vi "serialization test.vi"() -> ()   [LabVIEW 2013, in "std eng tests.lvlib"]
uses:
  std eng tests.lvlib
  Runtime/Standard Engine Runtime.lvclass
  <vilib>/NI/Tag Bus Module Framework/channel/channel classification.ctl
  <vilib>/NI/Tag Bus/tag/Data Type.ctl
  Configuration/Module Decimation.ctl
  Configuration/Supported Timing Sources.ctl
  testmodule/execution/testmod runtime.lvclass
  testmodule/configuration/testmod configuration.lvclass
  Configuration/Module Error Configuration.ctl
  Configuration/Error Actions By Category.ctl
  <vilib>/NI/Tag Bus Module Framework/runtime/error classification.ctl
  Configuration/Error Actions.ctl
  Configuration/timing reporting tags.ctl
  Configuration/Standard Engine Configuration.lvclass
  Configuration/Standard Engine Configuration.lvclass/Standard Engine Configuration.ctl
  <vilib>/NI/Tag Bus/tag/tag descriptor.lvclass
  Configuration/Write Timing Source Type.vi
  Configuration/Read Master Timing Module.vi
  Configuration/Read Module Specific Configuration.vi
  Configuration/Read Processor.vi
  Configuration/Read timing policy.vi
  Configuration/Read Timing Source Type.vi
  Configuration/Write Timing Source dt.vi
  Configuration/Find Module Specific Config.vi
  <vilib>/Utility/error.llb/Error Cluster From Error Code.vi
  <vilib>/NI/Configuration Framework/error generator.vi
  Configuration/Read Timing Source dt.vi
  <vilib>/NI/Tag Bus Module Framework/channel/TBM channel.lvclass
  <vilib>/NI/Module Execution Interface/Engine Configuration/engine configuration.lvclass
  <vilib>/NI/Tag Bus Module Framework/runtime/TBM module execution interface.lvclass
panel:
  out "Array":T1(array[cluster])
  out "x = y?":T2(array[cluster])
  out "serialization ok 7":bool
  out "serialization ok 6":bool
  out "serialization ok 5":bool
  out "serialization ok 4":bool
  out "serialization ok 3":bool
  out "serialization ok 2":bool
  out "serialization ok":bool
  out "errrrr":errorcluster
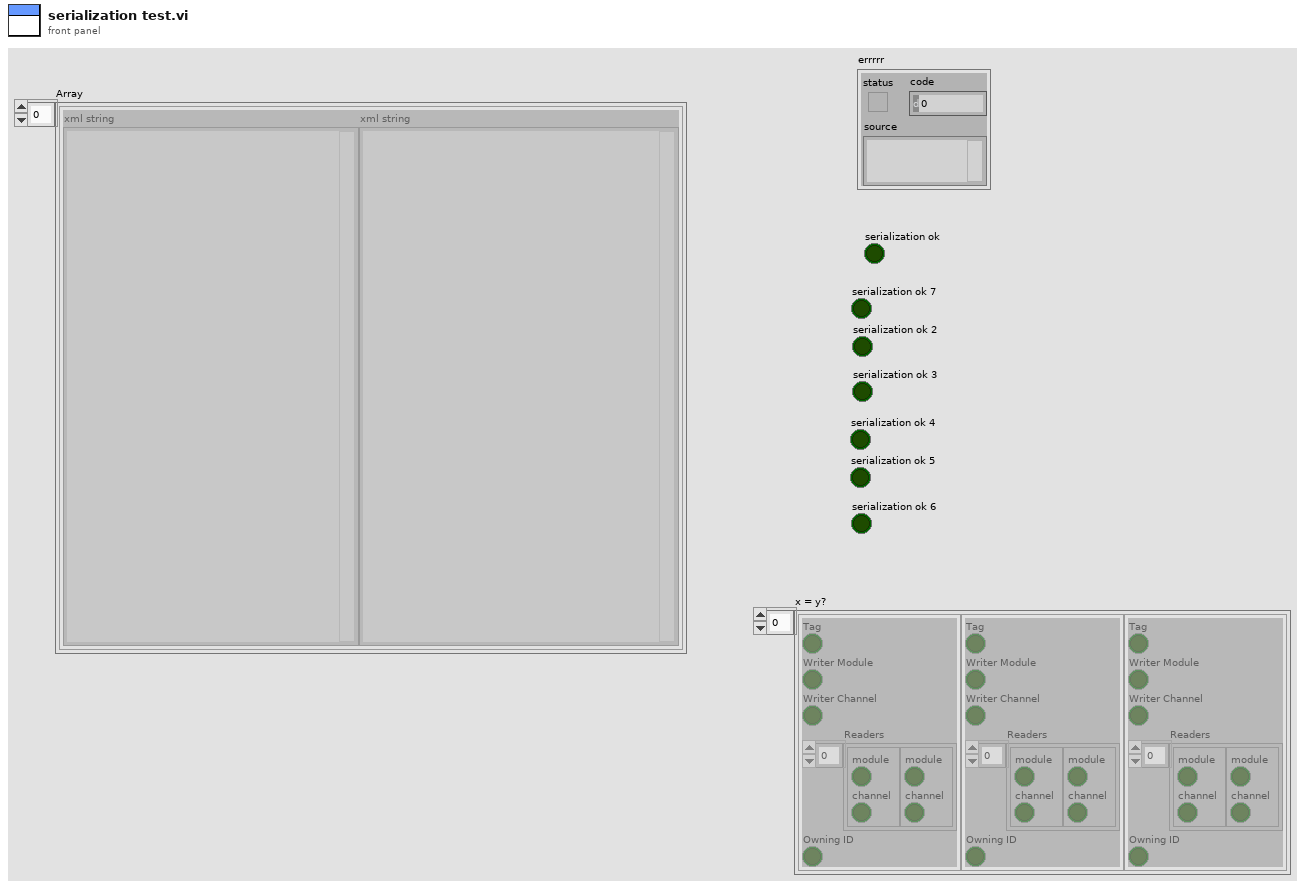
[diagram p1: front panel]
types:
  T1 = cluster{"xml string":string, "xml string":string}[]
  T2 = cluster{"Tag":bool, "Writer Module":bool, "Writer Channel":bool, "Readers":cluster{"module":bool, "channel":bool}[], "Owning ID":bool}[]
  T3 = typedef "Standard Engine Configuration.lvclass/timing reporting tags.ctl" = cluster{"late index (bool)":string, "late count index (U32)":string, "current dt ns(U64)":string}
  T4 = typedef "tag bus.lvlib/tag descriptor.lvclass/Data Type.ctl" = enum16{"Double", "Single", "I64", "I32", "I16", "I8", "U64", "U32", "U16", "U8", "Boolean", "String", "Array of Double", "Array of Single", "Array of I64", "Array of I32", "Array of I16", "Array of I8", "Array of U64", "Array of U32", "Array of U16", "Array of U8", "Array of Boolean", "Array of String"}
  T5 = typedef "TBM channel.lvclass/channel classification.ctl" = enum16{"input data", "output data", "processing parameter", "processing result"}
  T6 = typedef "Standard Engine Configuration.lvclass/Error Actions By Category.ctl" = cluster{"error classification":T7, "Error Actions":T8[]}
  T7 = typedef "TBM module execution interface.lvclass/error classification.ctl" = enum16{"unknown", "none", "trivial", "recoverable", "critical"}
  T8 = typedef "Standard Engine Configuration.lvclass/Error Actions.ctl" = enum16{"Clear", "Notify", "Stop Component", "Stop Engine", "Safe State", "Attempt Recovery"}
  T9 = typedef "Standard Engine Configuration.lvclass/Module Error Configuration.ctl" = cluster{"Module Error Configuration":T6[]}
  T10 = typedef "Standard Engine Configuration.lvclass/Supported Timing Sources.ctl" = enum16{"Use Module Timing Source", "1 kHz Clock", "1 MHz Clock", "Synchronize to Scan Engine"}
  T11 = typedef "Standard Engine Configuration.lvclass/Module Decimation.ctl" = cluster{"Decimation":u16, "Offset":u16}
  T12 = typedef "engine configuration.lvclass/Tag Info.ctl" = cluster{"Tag":refnum<class "tag descriptor.lvclass">, "Writer Module":string, "Writer Channel":string, "Readers":cluster{"module":string, "channel":string}[], "Owning ID":string}
  T13 = typedef "Standard Engine Configuration.lvclass/Module Specific Configuration.ctl" = cluster{"Module ID":string, "Module Decimation":T11, "Module Error Configuration":T9, "execution order priority":i32, "async?":bool, "error tag":string}
  T14 = typedef "Standard Engine Configuration.lvclass/timing policy.ctl" = enum16{"strict determinism", "nonblocking", "nondeterministic inline"}
  T15 = cluster{"xml string":string, "xml string":string}
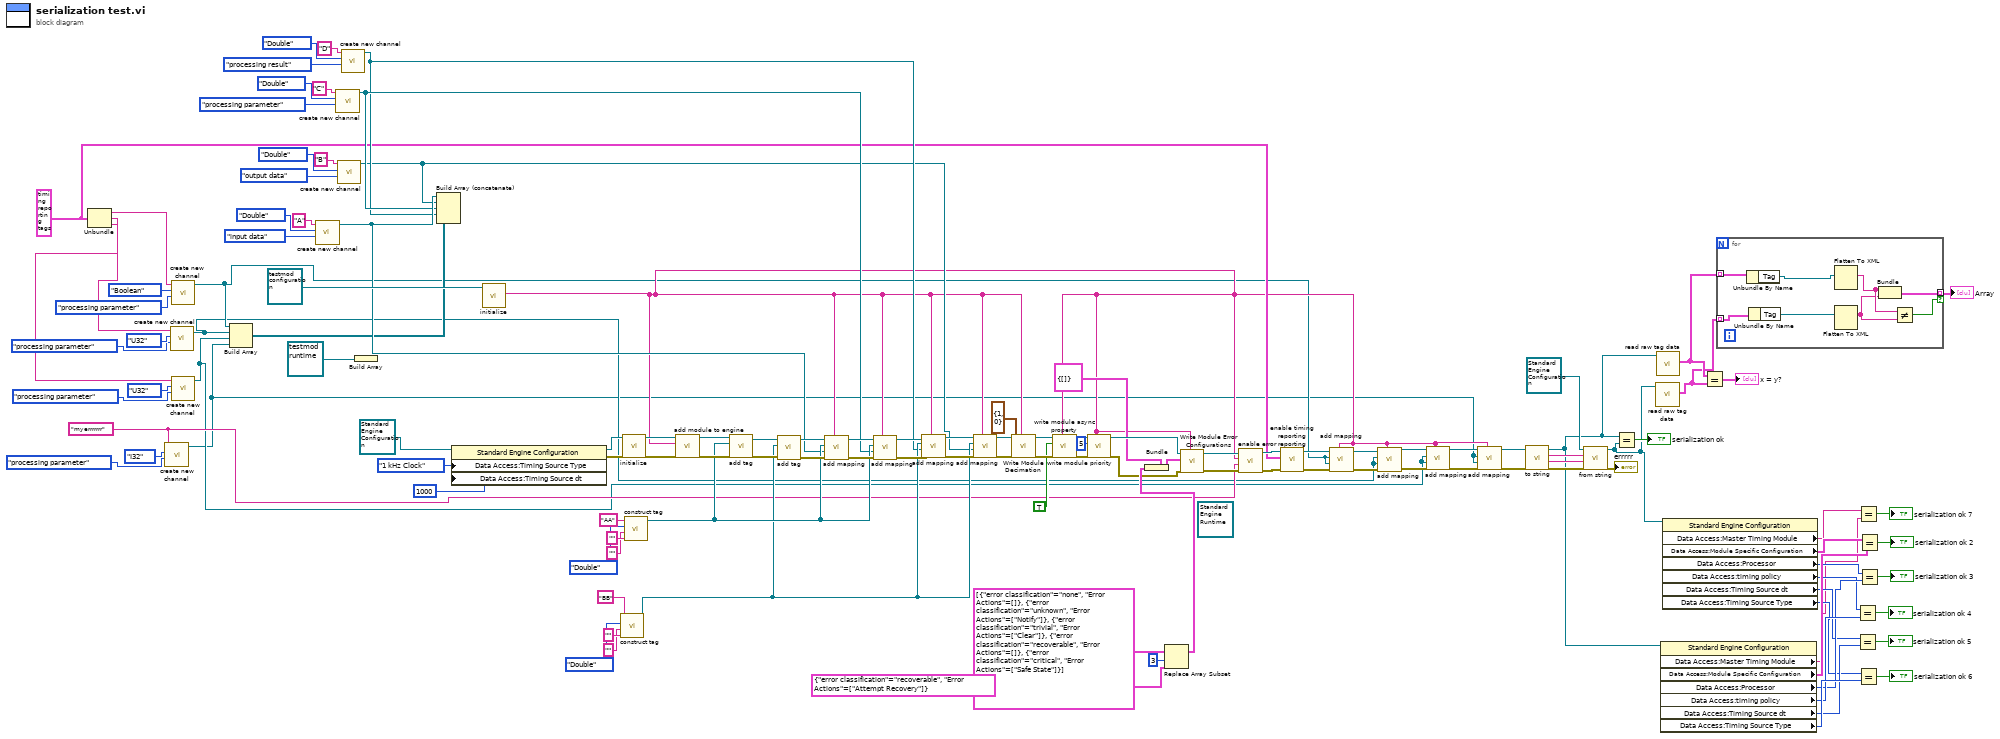
[diagram p0: block diagram]
diagram:
  w46 = T3 {"late index (bool)"="late", "late count index (U32)"="lcount", "current dt ns(U64)"="dt"} ("timing reporting")
  w47 = "myerrrrrrr" ("channel name")
  (unwired) refnum<class "Standard Engine Runtime.lvclass"> refnum ("Standard Engine Runtime")
  n1 = Unbundle(w46) -> ("late index (bool)"=w53:string, "late count index (U32)"=w52:string, "current dt ns(U64)"=w51:string)
  n2 = call <vilib>:"create new channel.vi"("channel classification"=channel_classification."processing parameter", "data type"=Data_Type."I32", "channel name"=w47) -> ("channel"=w33:refnum<class "TBM channel.lvclass">)  [unwired: 8 in]
  n3 = call <vilib>:"create new channel.vi"("channel classification"=channel_classification."processing parameter", "data type"=Data_Type."U32", "channel name"=w52) -> ("channel"=w35:refnum<class "TBM channel.lvclass">)  [unwired: 8 in]
  n4 = call <vilib>:"create new channel.vi"("channel classification"=channel_classification."processing parameter", "data type"=Data_Type."Boolean", "channel name"=w53) -> ("channel"=w36:refnum<class "TBM channel.lvclass">)  [unwired: 8 in]
  n5 = call <vilib>:"create new channel.vi"("channel classification"=channel_classification."processing parameter", "data type"=Data_Type."U32", "channel name"=w51) -> ("channel"=w34:refnum<class "TBM channel.lvclass">)  [unwired: 8 in]
  n6 = Build Array(w36, w35, w34, w33) -> (w48:refnum<class "TBM channel.lvclass">[])
  n7 = call <vilib>:"create new channel.vi"("channel classification"=channel_classification."input data", "data type"=Data_Type."Double", "channel name"="A") -> ("channel"=w75:refnum<class "TBM channel.lvclass">)  [unwired: 8 in]
  n8 = call <vilib>:"create new channel.vi"("channel classification"=channel_classification."processing parameter", "data type"=Data_Type."Double", "channel name"="C") -> ("channel"=w74:refnum<class "TBM channel.lvclass">)  [unwired: 8 in]
  n9 = call <vilib>:"create new channel.vi"("channel classification"=channel_classification."output data", "data type"=Data_Type."Double", "channel name"="B") -> ("channel"=w72:refnum<class "TBM channel.lvclass">)  [unwired: 8 in]
  n10 = call <vilib>:"create new channel.vi"("channel classification"=channel_classification."processing result", "data type"=Data_Type."Double", "channel name"="D") -> ("channel"=w73:refnum<class "TBM channel.lvclass">)  [unwired: 8 in]
  n11 = Build Array(refnum<class "testmod runtime.lvclass"> refnum ("CVT runtime")) -> ()  [unwired: 1 out]
  n12 = Build Array (concatenate)(w75, w72, w74, w73, w48) -> ()  [unwired: 1 out]
  n13 = property class="Standard Engine Configuration"(reference=refnum<class "Standard Engine Configuration.lvclass"> refnum ("Standard Engine Configuration"), "Data Access:Timing Source Type"=Supported_Timing_Sources."1 kHz Clock" ("Timing Source Type"), "Data Access:Timing Source dt"=u32 1000 ("Timing Source dt")) -> (reference out=w104:refnum<class "Standard Engine Configuration.lvclass">, error out=w106:errorcluster)  [unwired: 1 in]
  n14 = call-dynamic "initialize.vi"("configuration in"=refnum<class "testmod configuration.lvclass"> refnum ("CVT configuration")) -> ("identifier"=w37:string)  [unwired: 8 in, 2 out]
  n15 = call <vilib>:"construct tag.vi"("raw default"="", "metadata"="", "data type"=Data_Type."Double", "name"="BB") -> ("system tag out"=w76:refnum<class "tag descriptor.lvclass">)  [unwired: 6 in, 1 out]
  n16 = call-dynamic "initialize.vi"("error in"=w106, "configuration in"=w104) -> ("error out"=w117:errorcluster, "configuration out"=w116:refnum<class "Standard Engine Configuration.lvclass">)  [unwired: 7 in, 1 out]
  n17 = call <vilib>:"construct tag.vi"("raw default"="", "metadata"="", "data type"=Data_Type."Double", "name"="AA") -> ("system tag out"=w77:refnum<class "tag descriptor.lvclass">)  [unwired: 6 in, 1 out]
  n18 = call-dynamic "add module to engine.vi"("error in"=w117, "module ID"=w37, "Standard Engine Configuration in"=w116) -> ("error out"=w119:errorcluster, "Standard Engine Configuration out"=w118:refnum<class "Standard Engine Configuration.lvclass">)  [unwired: 7 in]
  n19 = call <vilib>:"add tag.vi"("error in"=w119, "tag descriptor"=w77, "engine configuration in"=w118) -> ("error out"=w92:errorcluster, "engine configuration out"=w93:refnum<class "Standard Engine Configuration.lvclass">)  [unwired: 7 in]
  n20 = call <vilib>:"add tag.vi"("error in"=w92, "tag descriptor"=w76, "engine configuration in"=w93) -> ("error out"=w91:errorcluster, "engine configuration out"=w79:refnum<class "Standard Engine Configuration.lvclass">)  [unwired: 7 in]
  n21 = call <vilib>:"add mapping.vi"("owner ID"=w37, "error in"=w91, "channel"=w75, "tag descriptor"=w77, "engine configuration"=w79) -> ("error out"=w80:errorcluster, "engine configuration out"=w78:refnum<class "Standard Engine Configuration.lvclass">)  [unwired: 5 in]
  n22 = call <vilib>:"add mapping.vi"("owner ID"=w37, "error in"=w80, "channel"=w74, "tag descriptor"=w77, "engine configuration"=w78) -> ("error out"=w82:errorcluster, "engine configuration out"=w81:refnum<class "Standard Engine Configuration.lvclass">)  [unwired: 5 in]
  n23 = call <vilib>:"add mapping.vi"("owner ID"=w37, "error in"=w82, "channel"=w73, "tag descriptor"=w76, "engine configuration"=w81) -> ("error out"=w121:errorcluster, "engine configuration out"=w120:refnum<class "Standard Engine Configuration.lvclass">)  [unwired: 5 in]
  n24 = call <vilib>:"add mapping.vi"("owner ID"=w37, "error in"=w121, "channel"=w72, "tag descriptor"=w76, "engine configuration"=w120) -> ("error out"=w112:errorcluster, "engine configuration out"=w113:refnum<class "Standard Engine Configuration.lvclass">)  [unwired: 5 in]
  n25 = call "Write Module Decimation.vi"("Module ID"=w37, "error in"=w112, "Module Decimation"=T11 {"Decimation"=1, "Offset"=0}, "Standard Engine Repo Data in"=w113) -> ("error out"=w114:errorcluster, "Standard Engine Repo Data out"=w115:refnum<class "Standard Engine Configuration.lvclass">)  [unwired: 6 in]
  n26 = call "write module async property.vi"("Module ID"=w37, "error in"=w114, "async?"=TRUE, "Standard Engine Repo Data in"=w115) -> ("error out"=w111:errorcluster, "Standard Engine Repo Data out"=w110:refnum<class "Standard Engine Configuration.lvclass">)  [unwired: 6 in]
  n27 = call "write module priority.vi"("Module ID"=w37, "error in"=w111, "execution order priority"=5, "Standard Engine Repo Data in"=w110) -> ("error out"=w60:errorcluster, "Standard Engine Repo Data out"=w71:refnum<class "Standard Engine Configuration.lvclass">)  [unwired: 6 in]
  n28 = Replace Array Subset(array=T6[] [{"error classification"=enum."none", "Error Actions"=[]}, {"error classification"=enum."unknown", "Error Actions"=[enum."Notify"]}, {"error classification"=enum."trivial", "Error Actions"=[enum."Clear"]}, {"error classification"=enum."recoverable", "Error Actions"=[]}, {"error classification"=enum."critical", "Error Actions"=[enum."Safe State"]}] ("Module Error Configuration"), new element=T6 {"error classification"=enum."recoverable", "Error Actions"=[enum."Attempt Recovery"]} ("Error Actions By Category"), index=3) -> (w67:T6[])
  n29 = Bundle(cluster=T9 {"Module Error Configuration"=[]} ("Module Error Configuration"), "Module Error Configuration"=w67) -> (w69:T9)
  n30 = call "Write Module Error Configurations.vi"("Module ID"=w37, "error in"=w60, "Module Error Configuration"=w69, "Standard Engine Repo Data in"=w71) -> ("error out"=w61:errorcluster, "Standard Engine Repo Data out"=w64:refnum<class "Standard Engine Configuration.lvclass">)  [unwired: 6 in]
  n31 = call "enable error reporting.vi"("error in"=w61, "tag"=w47, "module ID"=w37, "Standard Engine Configuration in"=w64) -> ("error out"=w62:errorcluster, "Standard Engine Configuration out"=w63:refnum<class "Standard Engine Configuration.lvclass">)  [unwired: 6 in]
  n32 = call "enable timing reporting.vi"("error in"=w62, "timing reporting"=w46, "Standard Engine Configuration in"=w63) -> ("error out"=w38:errorcluster, "Standard Engine Configuration out"=w39:refnum<class "Standard Engine Configuration.lvclass">)  [unwired: 7 in]
  n33 = call <vilib>:"add mapping.vi"("owner ID"=w37, "error in"=w38, "channel"=w36, "tag descriptor"=w36, "engine configuration"=w39) -> ("error out"=w44:errorcluster, "engine configuration out"=w45:refnum<class "Standard Engine Configuration.lvclass">)  [unwired: 5 in]
  n34 = call <vilib>:"add mapping.vi"("owner ID"=w37, "error in"=w44, "channel"=w35, "tag descriptor"=w35, "engine configuration"=w45) -> ("error out"=w42:errorcluster, "engine configuration out"=w43:refnum<class "Standard Engine Configuration.lvclass">)  [unwired: 5 in]
  n35 = call <vilib>:"add mapping.vi"("owner ID"=w37, "error in"=w42, "channel"=w34, "tag descriptor"=w34, "engine configuration"=w43) -> ("error out"=w40:errorcluster, "engine configuration out"=w41:refnum<class "Standard Engine Configuration.lvclass">)  [unwired: 5 in]
  n36 = call <vilib>:"add mapping.vi"("owner ID"=w37, "error in"=w40, "channel"=w33, "tag descriptor"=w33, "engine configuration"=w41) -> ("error out"=w31:errorcluster, "engine configuration out"=w30:refnum<class "Standard Engine Configuration.lvclass">)  [unwired: 5 in]
  n37 = call-dynamic "to string.vi"("error in"=w31, "Standard Engine Repo Data in"=w30) -> ("error out"=w32:errorcluster, "data"=w28:string, "version"=w29:string, "Standard Engine Repo Data out"=w5:refnum<class "Standard Engine Configuration.lvclass">)  [unwired: 6 in]
  n38 = call-dynamic "from string.vi"("error in"=w32, "data"=w28, "version"=w29, "Standard Engine Repo Data in"=refnum<class "Standard Engine Configuration.lvclass"> refnum ("Standard Engine Configuration")) -> ("error out"=→"errrrr":errorcluster, "Standard Engine Repo Data out"=w6:refnum<class "Standard Engine Configuration.lvclass">)  [unwired: 6 in]
  n39 = Equal?(x=w5, y=w6) -> (x = y?=→"serialization ok":bool)
  n40 = call <vilib>:"read raw tag data.vi"("engine configuration in"=w6) -> ("raw tag data"=w2:T12[])  [unwired: 8 in, 2 out]
  n41 = call <vilib>:"read raw tag data.vi"("engine configuration in"=w5) -> ("raw tag data"=w3:T12[])  [unwired: 8 in, 2 out]
  n42 = property class="Standard Engine Configuration"(reference=w5) -> ("Data Access:Master Timing Module"=w7:string, "Data Access:Module Specific Configuration"=w15:T13[], "Data Access:Processor"=w16:i32, "Data Access:timing policy"=w17:T14, "Data Access:Timing Source dt"=w18:u32, "Data Access:Timing Source Type"=w19:T10)  [unwired: 1 in, 2 out]
  n43 = property class="Standard Engine Configuration"(reference=w6) -> ("Data Access:Master Timing Module"=w8:string, "Data Access:Module Specific Configuration"=w14:T13[], "Data Access:Processor"=w13:i32, "Data Access:timing policy"=w12:T14, "Data Access:Timing Source dt"=w11:u32, "Data Access:Timing Source Type"=w10:T10)  [unwired: 1 in, 2 out]
  n44 = Equal?(x=w3, y=w2) -> (x = y?=→"x = y?":T2)
  n45 = for {
    tunnel: w3 -> [w135] mode=indexing
    tunnel: w2 -> [w134] mode=indexing
    tunnel: [w131] -> w1 mode=indexing if=w128
    n46 = Unbundle By Name(w135) -> ("Tag"=w133:refnum<class "tag descriptor.lvclass">)
    n47 = Unbundle By Name(w134) -> ("Tag"=w132:refnum<class "tag descriptor.lvclass">)
    n48 = Flatten To XML(anything=w133) -> (xml string=w130:string)
    n49 = Flatten To XML(anything=w132) -> (xml string=w129:string)
    n50 = Bundle("xml string"=w130, "xml string"=w129) -> (w131:T15)  [unwired: 1 in]
    n51 = Not Equal?(x=w130, y=w129) -> (x != y?=w128:bool)
  }
  "Array" <- w1
  n52 = Equal?(x=w12, y=w17) -> (x = y?=→"serialization ok 4":bool)
  n53 = Equal?(x=w11, y=w18) -> (x = y?=→"serialization ok 5":bool)
  n54 = Equal?(x=w8, y=w7) -> (x = y?=→"serialization ok 7":bool)
  n55 = Equal?(x=w10, y=w19) -> (x = y?=→"serialization ok 6":bool)
  n56 = Equal?(x=w14, y=w15) -> (x = y?=→"serialization ok 2":bool)
  n57 = Equal?(x=w13, y=w16) -> (x = y?=→"serialization ok 3":bool)
